vi "TBM.MoveFrontpanel.vi"(6 "VI lower corner?":bool, 8 "error in (no error)":errorcluster, 9 "VI right corner?":bool, 10 "Screen Position":cluster{"X":i16, "Y":i16}, 11 "VI in":refnum<vi>) -> (0 "error out":errorcluster, 3 "VI out":refnum<vi>)   [LabVIEW 2013, in "ToolbarMenu.lvlib"]
uses:
  ToolbarMenu.lvlib
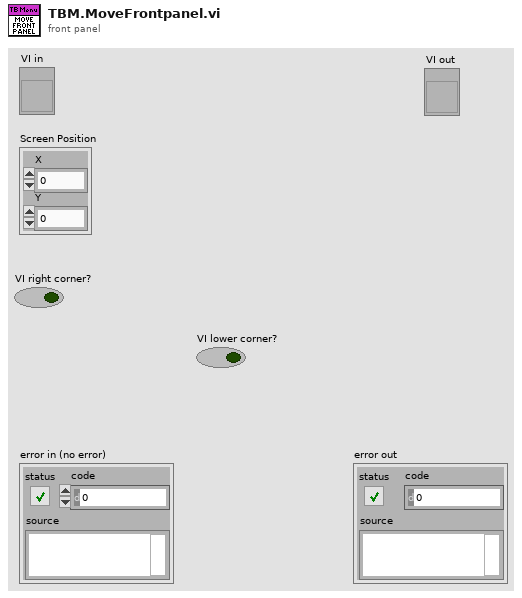
[diagram p1: front panel]
types:
  T1 = typedef "LVRectTypeDef.ctl" = cluster{"Left":i16, "Top":i16, "Right":i16, "Bottom":i16}
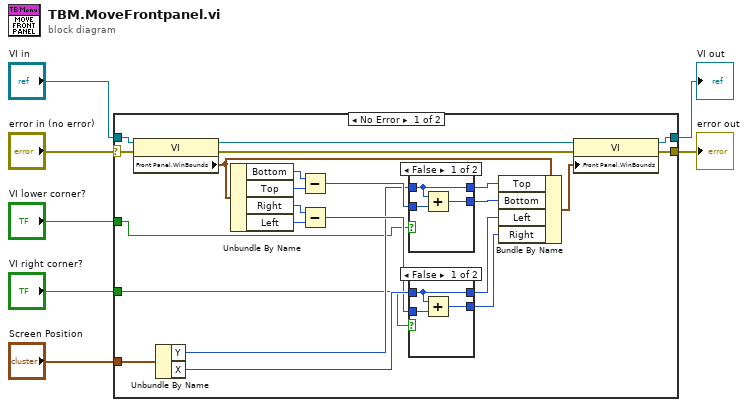
[diagram p0: block diagram]
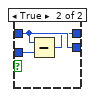
[diagram p2: hidden frame]
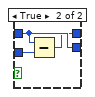
[diagram p3: hidden frame]
diagram:
  n1 = case shown="No Error" "error in (no error)" {
    selector: "error in (no error)" -> [w8 w44]
    tunnel: "VI in" -> [w29 w43]
    tunnel: [w27 w44] -> w6
    tunnel: [w25 w43] -> w5
    tunnel: "Screen Position" -> [w22 _]
    tunnel: "VI right corner?" -> [w10 _]
    tunnel: "VI lower corner?" -> [w9 _]
    frame No Error {
      n2 = property class="VI"(reference=w29, error in=w8) -> (reference out=w26:refnum<vi>, error out=w24:errorcluster, "Front Panel.WinBounds"=w20:T1)
      n3 = Unbundle By Name(w22) -> ("Y"=w18:i16, "X"=w23:i16)
      n4 = Unbundle By Name(w20) -> ("Bottom"=w17:i16, "Top"=w16:i16, "Right"=w15:i16, "Left"=w14:i16)
      n5 = Subtract(x=w17, y=w16) -> (x-y=w30:i16)
      n6 = Subtract(x=w15, y=w14) -> (x-y=w21:i16)
      n7 = case shown="False" w9 {
        tunnel: w18 -> [w37 w42]
        tunnel: w30 -> [w39 w41]
        tunnel: [w38 w42] -> w28
        tunnel: [w37 w40] -> w19
        frame False {
          n8 = Add(x=w37, y=w39) -> (x+y=w38:i16)
        }
        frame True {
          n9 = Subtract(x=w42, y=w41) -> (x-y=w40:i16)
        }
      }
      n10 = case shown="False" w10 {
        tunnel: [w33 w36] -> w12
        tunnel: w23 -> [w31 w36]
        tunnel: w21 -> [w32 w35]
        tunnel: [w31 w34] -> w13
        frame False {
          n11 = Add(x=w31, y=w32) -> (x+y=w33:i16)
        }
        frame True {
          n12 = Subtract(x=w36, y=w35) -> (x-y=w34:i16)
        }
      }
      n13 = Bundle By Name(cluster=w20, "Top"=w19, "Bottom"=w28, "Left"=w13, "Right"=w12) -> (w11:T1)
      n14 = property class="VI"(reference=w26, error in=w24, "Front Panel.WinBounds"=w11) -> (reference out=w25:refnum<vi>, error out=w27:errorcluster)
    }
    frame Error {
    }
  }
  "error out" <- w6
  "VI out" <- w5
